vi "String Subset Array.vi"(3 "Offset past End":i32[](array[numeric]), 4 "Start offset":i32[](array[numeric]), 5 "JSON":string) -> (1 "Subsets":string[](array[string]))   [LabVIEW 2024, in "JSONtext.lvlib"]
doc: "String subset between two offsets."
uses:
  JSONtext.lvlib
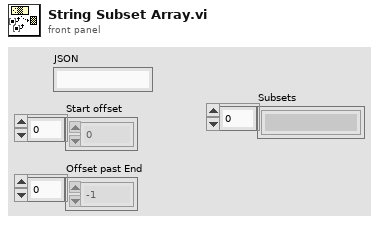
[diagram p1: front panel]
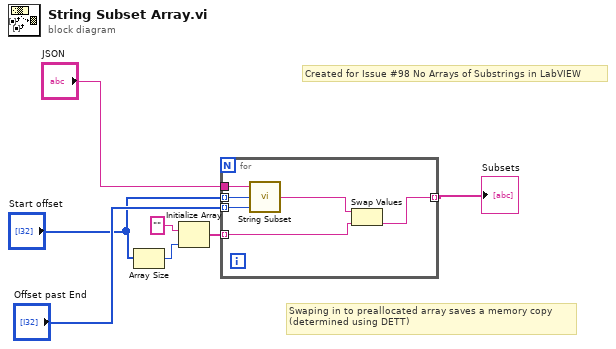
[diagram p0: block diagram]
diagram:
  # "Created for Issue #98 No Arrays of Substrings in LabVIEW"
  # "Swaping in to preallocated array saves a memory copy\n(determined using DETT)"
  n1 = Array Size(array="Start offset") -> (size(s)=w6:i32)
  n2 = Initialize Array("", w6) -> (w5:string[])
  n3 = for {
    tunnel: "Start offset" -> [w13] mode=indexing
    tunnel: "Offset past End" -> [w12] mode=indexing
    tunnel: "JSON" -> [w11]
    tunnel: [w8] -> w1 mode=indexing
    tunnel: w5 -> [w9] mode=indexing
    n4 = call "String Subset.vi"("Offset past End"=w12, "Start offset"=w13, "JSON"=w11) -> ("substring"=w10:string)  [unwired: 2 in]
    n5 = Swap Values(12:w10, 14:w9) -> (3:w8:string)  [unwired: 1 in, 1 out]
  }
  "Subsets" <- w1
